vi "Generic command handler.vi"(8 "error in (no error)":errorcluster, 10 "Message in":refnum<class "GenericMessage.lvclass">, 11 "Waveform in":refnum<class "Waveform.lvclass">) -> (0 "error out":errorcluster, 2 "value":string, 3 "Waveform out":refnum<class "Waveform.lvclass">)   [LabVIEW 2012, in "Waveform.lvclass"]
doc: "The generic_command_handler processes the command 'generic'. Commands which are not part of the predefined list of commands fall under the 'generic' command for special activity."
uses:
  Waveform.lvclass
  <vilib>/Distrio/Murmex/GenericMessage/GenericMessage.lvclass
  <vilib>/Distrio/Murmex/Murmex/Murmex.lvclass
  Waveform.lvclass/Waveform.ctl
  <vilib>/Distrio/Murmex/Message/Add or replace parameter.vi
  <vilib>/Distrio/Murmex/Message/Message.lvclass
panel:
  # "This method is called when the GENERIC\ntrigger is sent. \n\nOverride this method when your component needs to\nrespond to this trigger. \n\nCall parent for proper implementation"
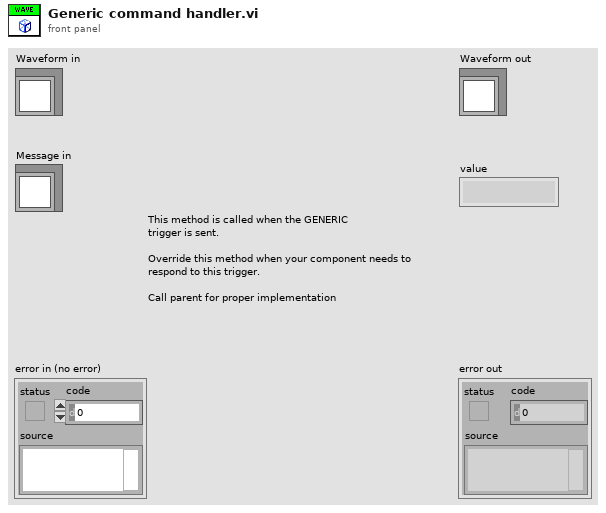
[diagram p1: front panel]
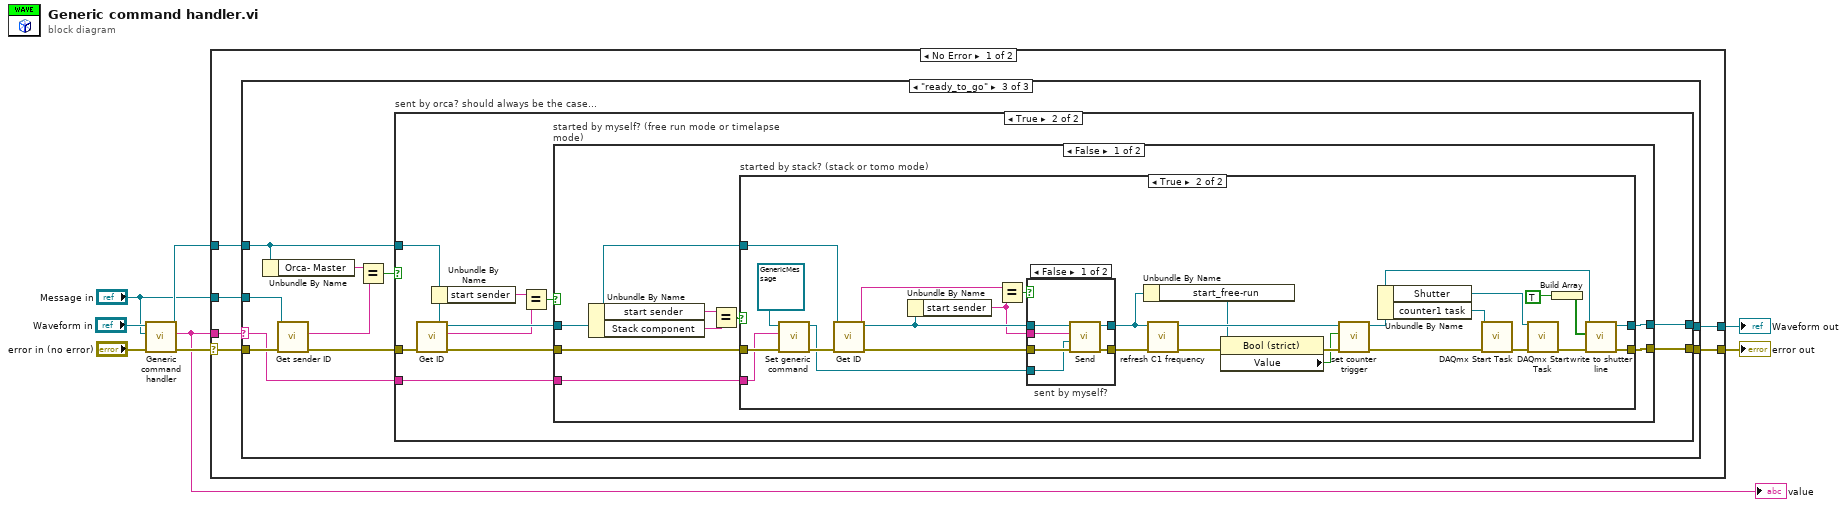
[diagram p0: block diagram]
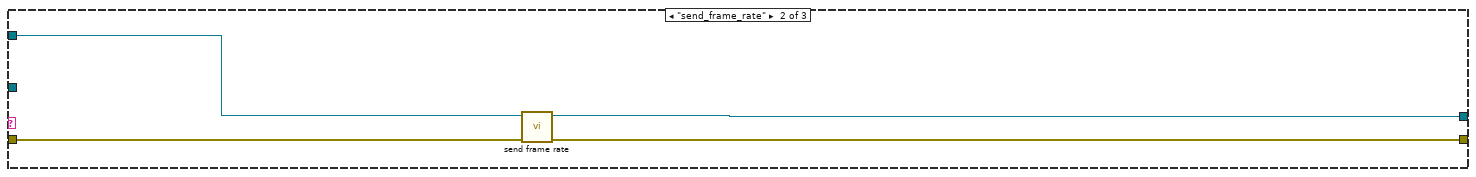
[diagram p3: hidden frame]
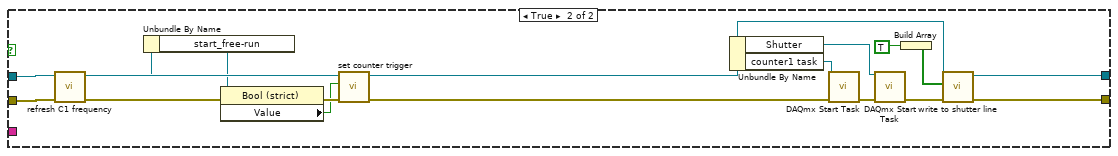
[diagram p7: hidden frame]
diagram:
  n1 = call-parent "Generic command handler.vi"("error in (no error)"="error in (no error)", "Message in"="Message in", "Murmex in"="Waveform in") -> ("error out"=w6:errorcluster, "value"=w2:string, "Murmex out"=w4:refnum<class "Waveform.lvclass">)  [unwired: 6 in]
  "value" <- w2
  n2 = case shown="No Error" w6 {
    selector: w6 -> [w14 w107]
    tunnel: [w11 w107] -> w5
    tunnel: w4 -> [w12 w106]
    tunnel: [w10 w106] -> w3
    tunnel: w2 -> [w13 _]
    tunnel: "Message in" -> [w9 _]
    frame No Error {
      n3 = case shown="\"ready_to_go\"" w13 {
        selector: w13 -> [_ _ w29]
        tunnel: w14 -> [w16 w20 w30]
        tunnel: w12 -> [w15 w19 w24]
        tunnel: [w16 w17 w28] -> w11
        tunnel: [w15 w18 w27] -> w10
        tunnel: w9 -> [_ _ w25]
        frame "False", Default {
        }
        frame "send_frame_rate" {
          n4 = call-dynamic "send frame rate.vi"("error in (no error)"=w20, "Waveform in"=w19) -> ("error out"=w17:errorcluster, "Waveform out"=w18:refnum<class "Waveform.lvclass">)  [unwired: 8 in]
        }
        frame "ready_to_go" {
          n5 = Unbundle By Name(w24) -> ("Orca- Master"=w23:string)
          n6 = call <vilib>:"Get sender ID.vi"("error in (no error)"=w30, "Message in"=w25) -> ("error out"=w26:errorcluster, "sender"=w21:string)  [unwired: 7 in, 1 out]
          n7 = Equal?(x=w23, y=w21) -> (x = y?=w22:bool)
          n8 = case "sent by orca? should always be the case..." shown="True" w22 {
            tunnel: w29 -> [_ w33]
            tunnel: [w32 w41] -> w28
            tunnel: [w31 w40] -> w27
            tunnel: w26 -> [w32 w42]
            tunnel: w24 -> [w31 w36]
            frame False {
            }
            frame True {
              n9 = call <vilib>:"Get ID.vi"("error in (no error)"=w42, "Murmex in"=w36) -> ("error out"=w37:errorcluster, "component id"=w34:string, "Murmex out"=w35:refnum<class "Waveform.lvclass">)  [unwired: 7 in]
              n10 = Unbundle By Name(w36) -> ("start sender"=w39:string)
              n11 = Equal?(x=w39, y=w34) -> (x = y?=w38:bool)
              n12 = case "started by myself? (free run mode or timelapse mode)" shown="False" w38 {
                tunnel: w37 -> [w47 w102]
                tunnel: [w46 w99] -> w41
                tunnel: [w45 w96] -> w40
                tunnel: w35 -> [w44 w95]
                tunnel: w33 -> [w43 _]
                frame False {
                  n13 = Unbundle By Name(w44) -> ("start sender"=w50:string, "Stack component"=w48:string)
                  n14 = Equal?(x=w50, y=w48) -> (x = y?=w49:bool)
                  n15 = case "started by stack? (stack or tomo mode)" shown="True" w49 {
                    tunnel: [w52 w58] -> w46
                    tunnel: [w51 w56] -> w45
                    tunnel: w47 -> [w52 w72]
                    tunnel: w44 -> [w51 w71]
                    tunnel: w43 -> [_ w70]
                    frame False {
                    }
                    frame True {
                      n16 = call <vilib>:"Set generic command.vi"("error in (no error)"=w72, "generic command"=w70, "GenericMessage in"=refnum<class "GenericMessage.lvclass"> refnum ("Distrio Murmex 1.2:GenericMessage")) -> ("error out"=w79:errorcluster, "GenericMessage out"=w73:refnum<class "GenericMessage.lvclass">)  [unwired: 7 in]
                      n17 = call <vilib>:"Get ID.vi"("error in (no error)"=w79, "Murmex in"=w71) -> ("error out"=w77:errorcluster, "component id"=w78:string, "Murmex out"=w75:refnum<class "Waveform.lvclass">)  [unwired: 7 in]
                      n18 = Unbundle By Name(w75) -> ("start sender"=w74:string)
                      n19 = Equal?(x=w78, y=w74) -> (x = y?=w76:bool)
                      n20 = case "sent by myself?" shown="False" w76 {
                        tunnel: w77 -> [w86 w87]
                        tunnel: [w85 w87] -> w57
                        tunnel: w75 -> [w84 w88]
                        tunnel: [w83 w88] -> w55
                        tunnel: w73 -> [w82 _]
                        tunnel: w74 -> [w81 _]
                        frame False {
                          n21 = call <vilib>:"Send.vi"("error in (no error)"=w86, "Message"=w82, "recipient"=w81, "Murmex in"=w84) -> ("error out"=w85:errorcluster, "Murmex out"=w83:refnum<class "Waveform.lvclass">)  [unwired: 6 in]
                        }
                        frame True {
                        }
                      }
                      n22 = Unbundle By Name(w55) -> ("start_free-run"=w60:refnum<vi>)
                      n23 = call-dynamic "refresh C1 frequency.vi"("error in (no error)"=w57, "Waveform in"=w55) -> ("error out"=w62:errorcluster, "Waveform out"=w64:refnum<class "Waveform.lvclass">)  [unwired: 8 in]
                      n24 = property class="Bool (strict)"(reference=w60, error in=w62) -> (error out=w61:errorcluster, "Value"=w59:bool)  [unwired: 1 out]
                      n25 = call-dynamic "set counter trigger.vi"("error in (no error)"=w61, "free run?"=w59, "Waveform in"=w64) -> ("error out"=w66:errorcluster, "Waveform out"=w63:refnum<class "Waveform.lvclass">)  [unwired: 7 in]
                      n26 = Unbundle By Name(w63) -> ("Shutter"=w69:refnum<k21>, "counter1 task"=w67:refnum<k21>)
                      n27 = call <vilib>:"DAQmx Start Task.vi"("task/channels in"=w67, "error in"=w66) -> ("error out"=w68:errorcluster)  [unwired: 12 in, 1 out]
                      n28 = call <vilib>:"DAQmx Start Task.vi"("task/channels in"=w69, "error in"=w68) -> ("error out"=w65:errorcluster)  [unwired: 12 in, 1 out]
                      n29 = Build Array(TRUE) -> (w53:bool[])
                      n30 = call-dynamic "write to shutter line.vi"("error in (no error)"=w65, "Output Array"=w53, "Waveform in"=w63) -> ("error out"=w58:errorcluster, "Waveform out"=w56:refnum<class "Waveform.lvclass">)  [unwired: 7 in]
                    }
                  }
                }
                frame True {
                  n31 = call-dynamic "refresh C1 frequency.vi"("error in (no error)"=w102, "Waveform in"=w95) -> ("error out"=w94:errorcluster, "Waveform out"=w98:refnum<class "Waveform.lvclass">)  [unwired: 8 in]
                  n32 = Unbundle By Name(w95) -> ("start_free-run"=w92:refnum<vi>)
                  n33 = property class="Bool (strict)"(reference=w92, error in=w94) -> (error out=w93:errorcluster, "Value"=w91:bool)  [unwired: 1 out]
                  n34 = call-dynamic "set counter trigger.vi"("error in (no error)"=w93, "free run?"=w91, "Waveform in"=w98) -> ("error out"=w101:errorcluster, "Waveform out"=w97:refnum<class "Waveform.lvclass">)  [unwired: 7 in]
                  n35 = Unbundle By Name(w97) -> ("Shutter"=w105:refnum<k21>, "counter1 task"=w103:refnum<k21>)
                  n36 = call <vilib>:"DAQmx Start Task.vi"("task/channels in"=w103, "error in"=w101) -> ("error out"=w104:errorcluster)  [unwired: 12 in, 1 out]
                  n37 = call <vilib>:"DAQmx Start Task.vi"("task/channels in"=w105, "error in"=w104) -> ("error out"=w100:errorcluster)  [unwired: 12 in, 1 out]
                  n38 = Build Array(TRUE) -> (w89:bool[])
                  n39 = call-dynamic "write to shutter line.vi"("error in (no error)"=w100, "Output Array"=w89, "Waveform in"=w97) -> ("error out"=w99:errorcluster, "Waveform out"=w96:refnum<class "Waveform.lvclass">)  [unwired: 7 in]
                }
              }
            }
          }
        }
      }
    }
    frame Error {
    }
  }
  "error out" <- w5
  "Waveform out" <- w3
